vi "KeyGray_normalbool.vi"(1 "OldVal":bool, 3 "引用":refnum<vi>) -> ()   [LabVIEW 2018]
panel:
  # "延时处理按键\n使其保持变灰50ms后恢复原状"
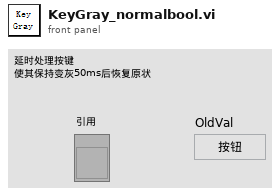
[diagram p1: front panel]
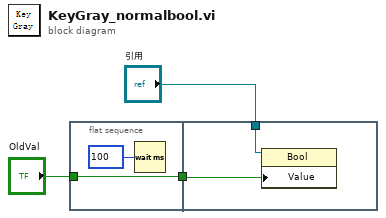
[diagram p0: block diagram]
diagram:
  n1 = flat-sequence {
    tunnel: "OldVal" -> [w5]
    tunnel: [w5] -> w2
    tunnel: w2 -> [w6]
    tunnel: "引用" -> [w7]
    frame #0 {
      n2 = Wait (ms)(milliseconds to wait=u32 100 ("等待时间（毫秒）")) -> ()  [unwired: 1 out]
    }
    frame #1 {
      n3 = property class="Bool"(reference=w7, "Value"=w6) -> ()  [unwired: 1 in, 2 out]
    }
  }
